vi "reconnect.vi"(8 "error in (no error)":errorcluster, 11 "SerialCommunicator in":refnum<class "SerialCommunicator.lvclass">) -> (0 "error out":errorcluster, 3 "SerialCommunicator out":refnum<class "SerialCommunicator.lvclass">)   [LabVIEW 2016, in "SerialCommunicator.lvclass"]
uses:
  SerialCommunicator.lvclass
  Communicator/Communicator.lvclass
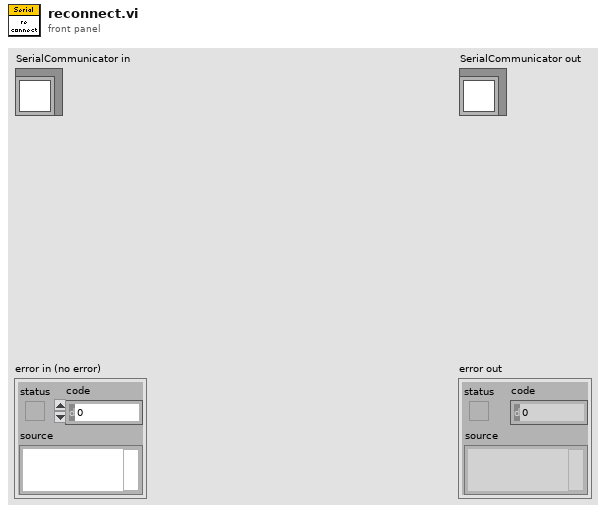
[diagram p1: front panel]
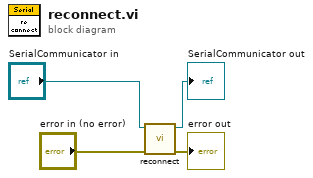
[diagram p0: block diagram]
diagram:
  n1 = call-parent "reconnect.vi"("error in (no error)"="error in (no error)", "Communicator in"="SerialCommunicator in") -> ("error out"=→"error out":errorcluster, "Communicator out"=→"SerialCommunicator out":refnum<class "SerialCommunicator.lvclass">)  [unwired: 8 in]
